vi "Error Query.vi"(8 "error in (no error)":errorcluster, 11 "Driver in":refnum<class "Driver.lvclass">) -> (0 "error out":errorcluster, 2 "read buffer":string, 3 "Driver out":refnum<class "Driver.lvclass">)   [LabVIEW 2023, in "Driver.lvlib" / "Driver.lvclass"]
uses:
  Driver.lvclass
  Driver.lvclass/Driver.ctl
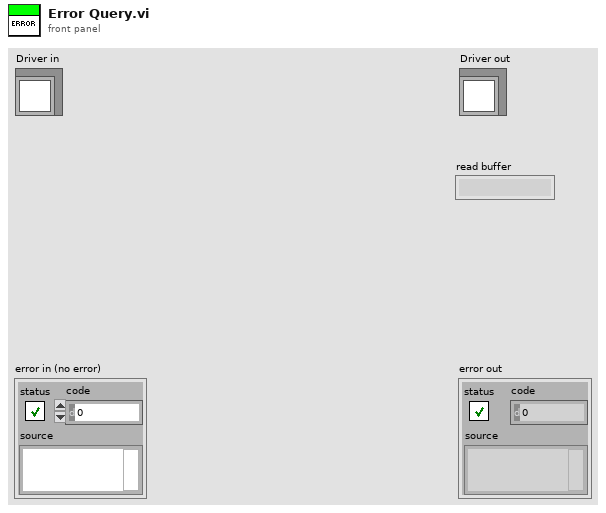
[diagram p1: front panel]
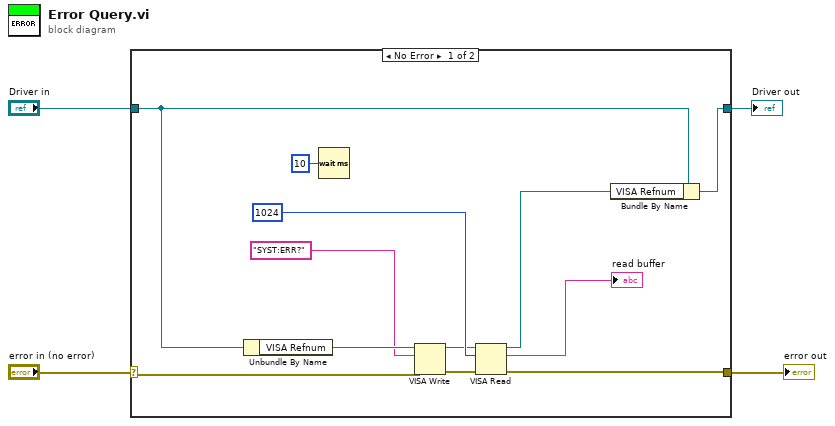
[diagram p0: block diagram]
diagram:
  n1 = case shown="No Error" "error in (no error)" {
    selector: "error in (no error)" -> [w11 w18]
    tunnel: [w10 w18] -> w3
    tunnel: [w8 w17] -> w1
    tunnel: "Driver in" -> [w9 w17]
    frame No Error {
      n2 = Unbundle By Name(w9) -> ("VISA Refnum"=w16:refnum<visa-resource-name>)
      n3 = Wait (ms)(milliseconds to wait=u32 10) -> ()  [unwired: 1 out]
      n4 = VISA Write(VISA resource name=w16, write buffer="SYST:ERR?", error in (no error)=w11) -> (VISA resource name out=w13:refnum<visa-resource-name>, error out=w14:errorcluster)  [unwired: 1 out]
      n5 = VISA Read(VISA resource name=w13, byte count=u32 1024, error in (no error)=w14) -> (VISA resource name out=w7:refnum<visa-resource-name>, read buffer=→"read buffer":string, error out=w10:errorcluster)  [unwired: 1 out]
      n6 = Bundle By Name(cluster=w9, "VISA Refnum"=w7) -> (w8:refnum<class "Driver.lvclass">)
    }
    frame Error {
    }
  }
  "error out" <- w3
  "Driver out" <- w1
